vi "Get Interface Count.vi"(8 "error in (no error)":errorcluster) -> (0 "error out":errorcluster, 3 "count":i32)   [LabVIEW 2025, in "Automotive Ethernet Bus Monitor UI.lvlib" / "lvwpcap.lvlib"]
doc: "This VI outputs the number of active ethernet interfaces in your computer."
uses:
  lvwpcap.lvlib
  lvwpcap.dll
panel:
  # "Select Help»Show Context Help and move the cursor over the VI icon to display help for this VI."
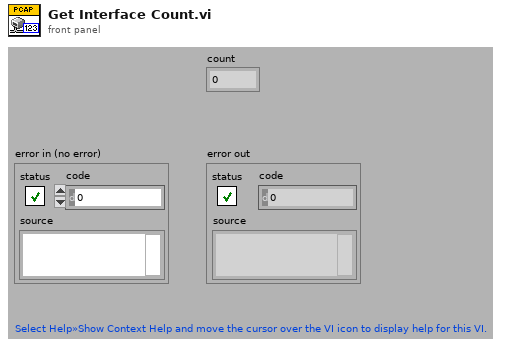
[diagram p1: front panel]
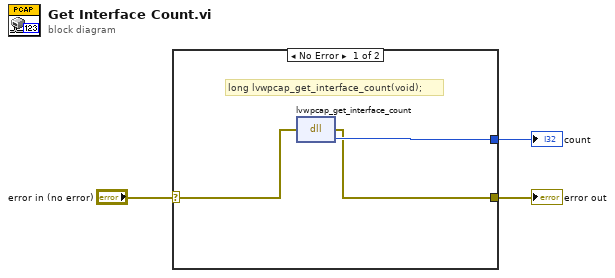
[diagram p0: block diagram]
diagram:
  n1 = case shown="No Error" "error in (no error)" {
    selector: "error in (no error)" -> [w5 w7]
    tunnel: [w4 w7] -> w2
    tunnel: [w6 _] -> w1
    frame No Error {
      # "long lvwpcap_get_interface_count(void);"
      n2 = dll-call lib="lvwpcap.*" fn="lvwpcap_get_interface_count"(error in=w5) -> (error out=w4:errorcluster, "return type"=w6:i32)  [unwired: 2 in, 1 out]
    }
    frame Error {
    }
  }
  "error out" <- w2
  "count" <- w1
